vi "Init.vi"(8 "Error In":errorcluster, 10 "IConfigure in":refnum<class "IConfigure.lvclass">=refnum, 11 "object in":refnum<class "Teledyne-T3AFG120.lvclass">=refnum) -> (0 "Error Out":errorcluster, 3 "object out":refnum<class "Teledyne-T3AFG120.lvclass">)   [LabVIEW 2023, in "Teledyne-T3AFG120.lvlib" / "Teledyne-T3AFG120.lvclass"]
uses:
  Teledyne-T3AFG120.lvclass
  interfaces/IConfigureViaUSB_interface/IConfigureViaUSB.lvclass
  IConfigure_interface/IConfigure.lvclass
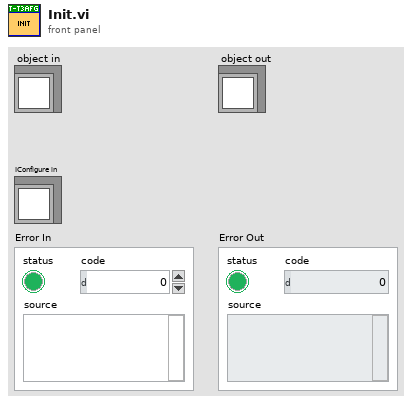
[diagram p1: front panel]
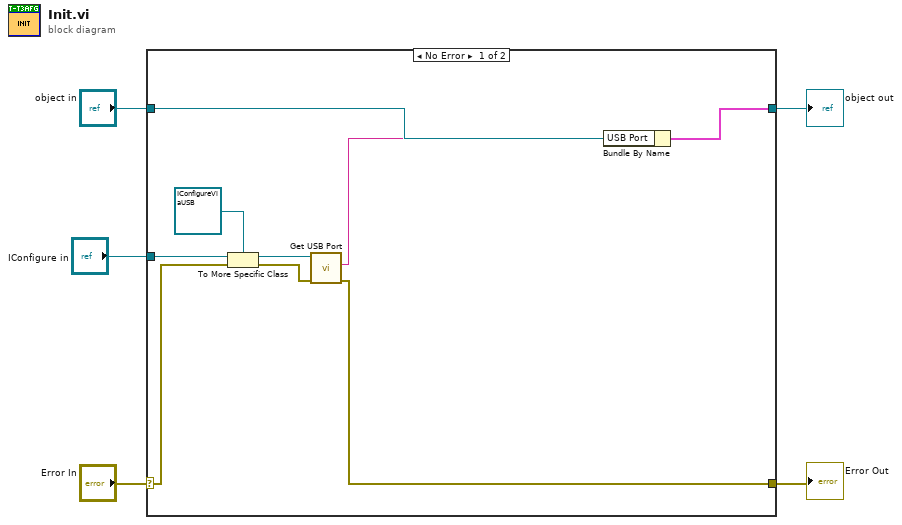
[diagram p0: block diagram]
diagram:
  n1 = case shown="No Error" "Error In" {
    selector: "Error In" -> [w12 w16]
    tunnel: [w7 w16] -> w4
    tunnel: [w8 w15] -> w2
    tunnel: "object in" -> [w14 w15]
    tunnel: "IConfigure in" -> [w13 _]
    frame No Error {
      n2 = To More Specific Class(target class=refnum<class "IConfigureViaUSB.lvclass"> refnum ("HAL.lvlib:IConfigureViaUSB"), reference=w13, error in=w12) -> (specific class reference=w10:refnum<class "IConfigureViaUSB.lvclass">, error out=w9:errorcluster)
      n3 = call-dynamic "Get USB Port.vi"("Error In"=w9, "object in"=w10) -> ("Error Out"=w7:errorcluster, "USB Port"=w6:string)  [unwired: 7 in, 1 out]
      n4 = Bundle By Name(cluster=w14, "USB Port"=w6) -> (w8:cluster{})
    }
    frame Error {
    }
  }
  "Error Out" <- w4
  "object out" <- w2
